vi "Inflation Camera.vi"(8 "error in (no error)":errorcluster, 9 "gui notifier":refnum<notifier>, 10 "error queue":refnum<queue>, 11 "cam notifier":refnum<notifier>) -> (0 "error out":errorcluster)   [LabVIEW 2020]
uses:
  Hardware/Sensors/Cameras/Camera.lvclass
  Main GUI Loop/Handler.ctl
  Hardware/Sensors/Cameras/Camera.lvclass/Camera.ctl
  Hardware/Read timestamp.vi
panel:
  out "current image":T1(plugin-control)
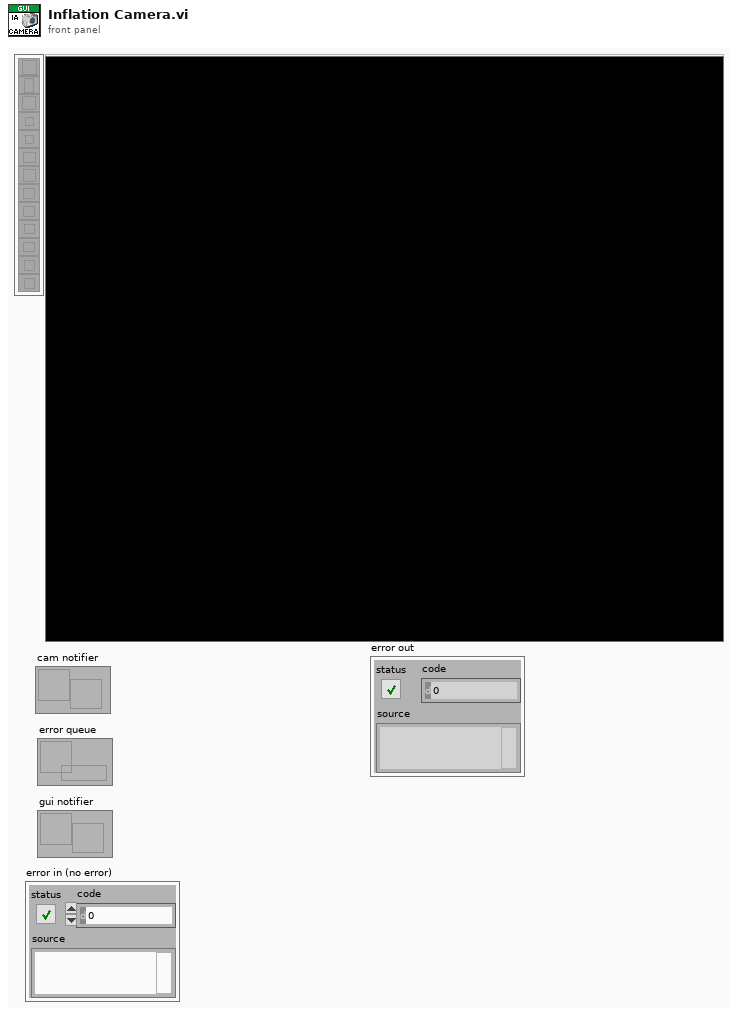
[diagram p1: front panel]
types:
  T1 = typedef "IMAQ Image.ctl" = refnum<image>
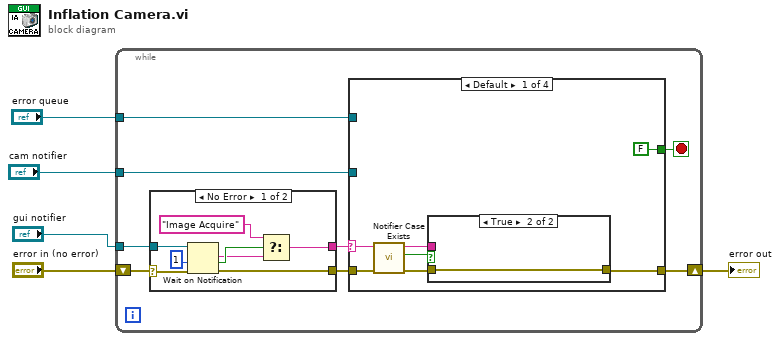
[diagram p0: block diagram]
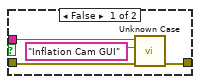
[diagram p2: hidden frame]
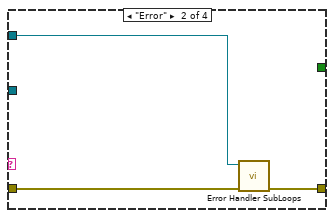
[diagram p3: hidden frame]
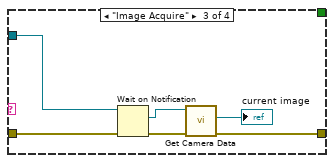
[diagram p4: hidden frame]
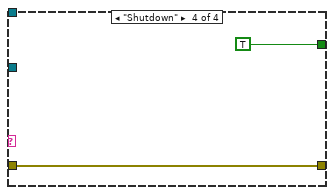
[diagram p5: hidden frame]
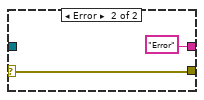
[diagram p6: hidden frame]
diagram:
  n1 = while {
    tunnel: "cam notifier" -> [w12]
    tunnel: "gui notifier" -> [w11]
    shift-right: [w8] -> w2
    shift-left: "error in (no error)" -> [w10]
    tunnel: "error queue" -> [w6]
    stop <- w13 stop-if-true
    n2 = case shown="No Error" w10 {
      selector: w10 -> [w41 w46]
      tunnel: w11 -> [w44 _]
      tunnel: [w43 w46] -> w9
      tunnel: [w37 "Error" ("gui msg")] -> w7
      frame No Error {
        n3 = Wait on Notification(notifier=w44, timeout in ms (-1)=1, error in (no error)=w41) -> (notification=w39:string, timed out?=w40:bool, error out=w43:errorcluster)  [unwired: 1 in, 1 out]
        n4 = Select(t="Image Acquire", s=w40, f=w39) -> (s? t:f=w37:string)
      }
      frame Error {
      }
    }
    n5 = case shown="Default" w7 {
      selector: w7 -> [w16 _ _ _]
      tunnel: [FALSE _ _ TRUE] -> w13
      tunnel: w12 -> [_ _ w31 _]
      tunnel: w9 -> [w18 w27 w30 w35]
      tunnel: [w19 w26 w29 w35] -> w8
      tunnel: w6 -> [_ w28 _ _]
      frame Default {
        n6 = call "Notifier Case Exists.vi"("error in (no error)"=w18, "case in"=w16) -> ("error out"=w17:errorcluster, "defined case?"=w14:bool, "case out"=w15:string)  [unwired: 7 in]
        n7 = case shown="True" w14 {
          tunnel: [w24 w25] -> w19
          tunnel: w17 -> [w22 w25]
          tunnel: w15 -> [w21 _]
          frame False {
            n8 = call "Unknown Case.vi"("error in (no error)"=w22, "source"="Inflation Cam GUI", "case"=w21) -> ("error out"=w24:errorcluster)  [unwired: 8 in]
          }
          frame True {
          }
        }
      }
      frame "Error" {
        n9 = call "Error Handler SubLoops.vi"("error in"=w27, "main gui queue"=w28) -> ("error out"=w26:errorcluster)  [unwired: 9 in]
      }
      frame "Image Acquire" {
        n10 = Wait on Notification(notifier=w31, error in (no error)=w30) -> (notification=w34:refnum<class "Camera.lvclass">, error out=w32:errorcluster)  [unwired: 2 in, 2 out]
        n11 = call "Get Camera Data.vi"("error in (no error)"=w32, "Camera in"=w34) -> ("error out"=w29:errorcluster, "image"=→"current image":T1)  [unwired: 5 in, 3 out]
      }
      frame "Shutdown" {
      }
    }
  }
  "error out" <- w2
